vi "Update Options.vi"(8 "error in (no error)":errorcluster, 10 "Options":string[](array[string]), 11 "Shared Options in":refnum<class "Shared Options.lvclass">) -> (0 "error out":errorcluster, 3 "Shared Options out":refnum<class "Shared Options.lvclass">)   [LabVIEW 2020, in "AutoComplete.lvlib" / "Shared Options.lvclass"]
uses:
  Shared Options.lvclass
  Shared Options.lvclass/Shared Options.ctl
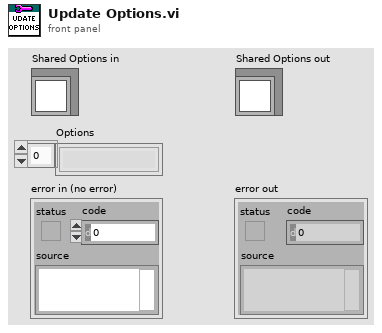
[diagram p1: front panel]
types:
  T1 = typedef "AutoComplete.lvlib/Options.ctl" = cluster{"Options":string[], "Allow Undefined Values":bool}
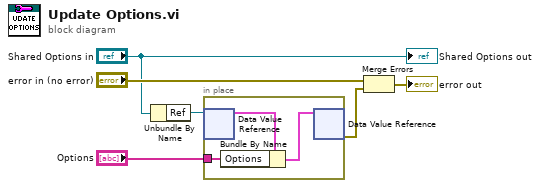
[diagram p0: block diagram]
diagram:
  n1 = Unbundle By Name("Shared Options in") -> ("Ref"=w4:refnum<data-value>)
  n2 = in-place {
    in-place-border: "Options" -> [w7]
    n3 = in-place-dvr #1(w4) -> (w9:T1)  [unwired: 1 out]
    n4 = Bundle By Name(cluster=w9, "Options"=w7) -> (w8:T1)
    n5 = in-place-dvr #1(w8) -> (w2:errorcluster)  [unwired: 1 out]
  }
  n6 = Merge Errors("error in (no error)", w2) -> (→"error out":errorcluster)
  "Shared Options out" <- "Shared Options in"
